vi "Analog TestCode.vi"(10 "?":string="String") -> (2 "String":string)   [LabVIEW 2014]
panel:
  out "Voltage For Analog":dbl
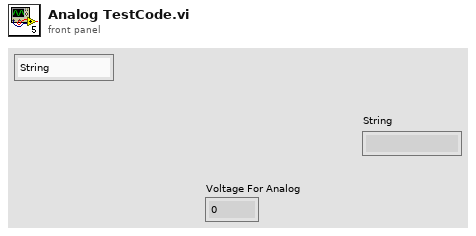
[diagram p1: front panel]
types:
  T1 = typedef "WPI_AnalogChannelDevRef.ctl" = cluster{"DevStatus":errorcluster, "Controller":T2, "Analog Channel":T3}
  T2 = typedef "FPGA_TypedefAnalogModule.ctl" = enum16{"Controller 1"}
  T3 = typedef "FPGA_AIChannel.ctl" = enum8{"AI 0", "AI 1", "AI 2", "AI 3", "AI MXP 0", "AI MXP 1", "AI MXP 2", "AI MXP 3", "Invalid"}
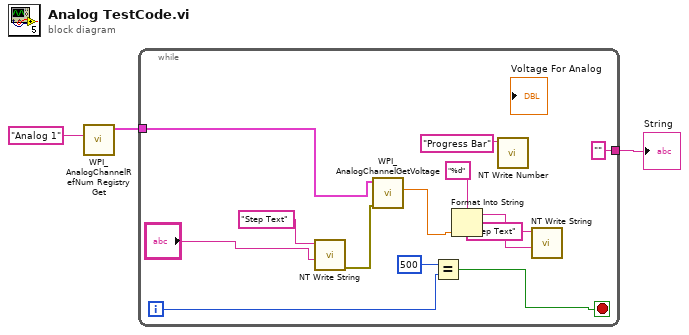
[diagram p0: block diagram]
diagram:
  n1 = call <vilib>:"WPI_AnalogChannelRefNum Registry Get.vi"("refnum name"="Analog 1") -> ("AIDeviceRef"=w1:T1)  [unwired: 9 in, 1 out]
  n2 = while {
    tunnel: ["" ("String")] -> w3
    tunnel: w1 -> [w10]
    i -> [w13]
    stop <- w12 stop-if-true
    n3 = call <vilib>:"NT Write String.vi"("String"="?", "Name"="Step Text" ("String")) -> ("error out"=w16:errorcluster)  [unwired: 9 in]
    n4 = call <vilib>:"WPI_AnalogChannelGetVoltage.vi"("error in (no error)"=w16, "AIDeviceRef"=w10) -> ("Voltage"=w9:dbl)  [unwired: 7 in, 2 out]
    n5 = Equal?(x=500, y=w13) -> (x = y?=w12:bool)
    n6 = Format Into String(format string="%d", w9) -> (resulting string=w7:string)  [unwired: 2 in, 1 out]
    n7 = call <vilib>:"NT Write Number.vi"("Name"="Progress Bar") -> ()  [unwired: 10 in, 1 out]
    n8 = call <vilib>:"NT Write String.vi"("String"=w7, "Name"="Step Text") -> ()  [unwired: 9 in, 1 out]
  }
  "String" <- w3
